vi "Sensor Pick Up v2.vi"   [LabVIEW 2020]
uses:
  Classes/Workspace/Pick Up Tool Area/Pick Up Tool Fixture.lvclass
  Classes/Routine/Pick and Place/Pick and Place Type.ctl
  Classes/Workspace/Component/Component Tray.lvclass
  Classes/Routine/Pick and Place/Pick and Place.lvclass
  Classes/Routine/Pick and Place/Pick and Place.lvclass/Pick and Place.ctl
  Classes/Routine/Pick and Place/Write Pick and Place Type.vi
  Classes/Controller/Controller.lvclass
types:
  T1 = typedef "Pick and Place.lvclass/Pick and Place Type.ctl" = enum16{"Primary Pick Up", "Secondary Pick Up", "Put Down All", "Pick Up All", "Put Down Secondary"}
  T2 = typedef "Controller.lvclass/Controllers.ctl" = cluster{"I-O.lvclass":refnum<class "I-O.lvclass">, "Dispenser.lvclass":refnum<class "Dispenser.lvclass">, "Gantry":refnum<k24>}
  T3 = typedef "Fixture.lvclass/Workspace.ctl" = cluster{"XYZTheta":dbl[], "Workspace Valve":i32, "Workspace Sensor":i32}
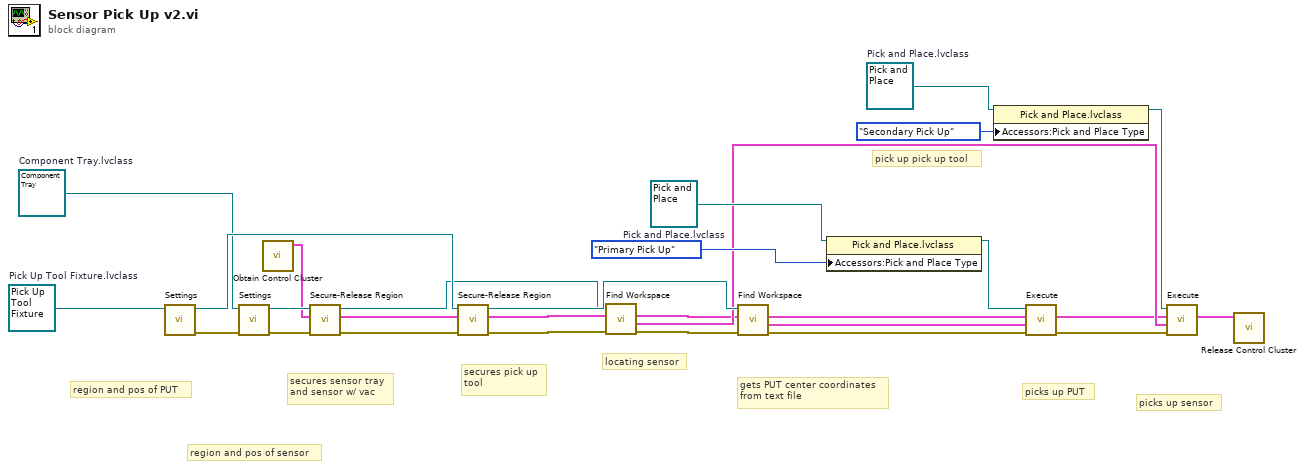
[diagram p0: block diagram]
diagram:
  w18 = refnum<class "Pick and Place.lvclass"> refnum  # Pick and Place.lvclass
  w1 = refnum<class "Component Tray.lvclass"> refnum  # Component Tray.lvclass
  w25 = refnum<class "Pick and Place.lvclass"> refnum  # Pick and Place.lvclass
  w28 = refnum<class "Pick Up Tool Fixture.lvclass"> refnum  # Pick Up Tool Fixture.lvclass
  # "picks up PUT"
  # "gets PUT center coordinates\nfrom text file"
  # "secures pick up\ntool"
  # "secures sensor tray \nand sensor w/ vac"
  # "region and pos of sensor"
  # "region and pos of PUT"
  # "locating sensor"
  # "picks up sensor"
  # "pick up pick up tool"
  n1 = call-dynamic "Settings.vi"("Workspace in"=w28) -> ("error out"=w13:errorcluster, "Workspace out"=w27:refnum<class "Pick Up Tool Fixture.lvclass">)  [unwired: 9 in]
  n2 = call-dynamic "Settings.vi"("error in (no error)"=w13, "Component in"=w1) -> ("error out"=w14:errorcluster, "Component out"=w20:refnum<class "Component Tray.lvclass">)  [unwired: 8 in]
  n3 = call "Obtain Control Cluster.vi"() -> ("Control Out"=w12:T2)  [unwired: 11 in]
  n4 = call-dynamic "Secure-Release Region.vi"("error in (no error)"=w14, "Control In"=w12, "Workspace in"=w20) -> ("error out"=w10:errorcluster, "Control Out"=w11:T2, "Workspace out"=w19:refnum<class "Component Tray.lvclass">)  [unwired: 6 in]
  n5 = call-dynamic "Secure-Release Region.vi"("error in (no error)"=w10, "Control In"=w11, "Fixture in"=w27) -> ("error out"=w9:errorcluster, "Control Out"=w7:T2, "Fixture out"=w26:refnum<class "Pick Up Tool Fixture.lvclass">)  [unwired: 6 in]
  n6 = call-dynamic "Find Workspace.vi"("error in (no error)"=w9, "Control In"=w7, "Component.lvclass"=w19) -> ("error out"=w8:errorcluster, "Workspace"=w15:T3, "Control Out"=w6:T2)  [unwired: 5 in, 1 out]
  n7 = call-dynamic "Find Workspace.vi"("Error In"=w8, "Control In"=w6, "Workspace In"=w26) -> ("Error Out"=w5:errorcluster, "Workspace Out"=w22:T3, "Control Out"=w21:T2)  [unwired: 5 in, 1 out]
  n8 = property class="Pick and Place.lvclass"(reference=w25, "Accessors:Pick and Place Type"=Pick_and_Place_Type."Primary Pick Up" ("Pick and Place Type")) -> (reference out=w23:refnum<class "Pick and Place.lvclass">)  [unwired: 1 in, 1 out]
  n9 = property class="Pick and Place.lvclass"(reference=w18, "Accessors:Pick and Place Type"=Pick_and_Place_Type."Secondary Pick Up" ("Pick and Place Type")) -> (reference out=w16:refnum<class "Pick and Place.lvclass">)  [unwired: 1 in, 1 out]
  n10 = call-dynamic "Execute.vi"("error in (no error)"=w5, "Workspace"=w22, "Cluster"=w21, "Pick and Place in"=w23) -> ("error out"=w4:errorcluster, "Control Out"=w3:T2)  [unwired: 5 in, 1 out]
  n11 = call-dynamic "Execute.vi"("error in (no error)"=w4, "Workspace"=w15, "Cluster"=w3, "Pick and Place in"=w16) -> ("Control Out"=w2:T2)  [unwired: 5 in, 2 out]
  n12 = call "Release Control Cluster.vi"("output cluster"=w2) -> ()  [unwired: 11 in]
